vi "Framework State.Get Active Plugins.vi"(11 "Framework State in":refnum<class "Framework State.lvclass">) -> (2 "Active Plugins":bool[](array[boolean]), 3 "Framework State out":refnum<class "Framework State.lvclass">)   [LabVIEW 2017, in "DSF Core.lvlib" / "Framework State.lvclass"]
uses:
  Framework State.lvclass
  Framework State.lvclass/Framework State.ctl
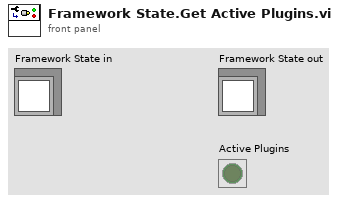
[diagram p1: front panel]
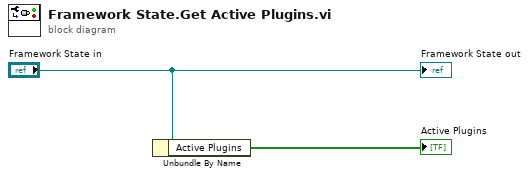
[diagram p0: block diagram]
diagram:
  n1 = Unbundle By Name("Framework State in") -> ("Active Plugins"=→"Active Plugins":bool[])
  "Framework State out" <- "Framework State in"
